vi "SkewedChi2Sampler.vi"(8 "error in":errorcluster caption="entrée d'erreur", 11 "SkewedChi2Sampler":T1={"skewedness"=1.0, "n_components"=100, "random_state"=-1} {"random_state" min=-1}) -> (0 "error out":errorcluster caption="sortie d'erreur", 3 "SkewedChi2Sampler.lvclass":refnum<class "SkewedChi2Sampler.lvclass">)   [LabVIEW 2020]
doc: "Approximates feature map of the “skewed chi-squared” kernel by Monte Carlo approximation of its Fourier transform.\n\nParameters :\n\n- skewedness : float\n“skewedness” parameter of the kernel. Needs to be cross-validated.\n\n- n_components : int\nnumber of Monte Carlo samples per original feature. Equals the dimensionality of the computed feature space.\n\n- random_state : int, RandomState instance or None, optional (default=None=-1)\nPseudo-random number generator to control the generation of the random weights and random offset when fitting the training data. Pass an int for reproducible output across multiple function calls. \n\nMethods : \n\n- Fit : Fit the model with X. Samples random projection according to n_features.\n\nParameters : X : array-like, shape (n_samples, n_features)\n Training data, where n_samples in the number of samples and n_features is the number of features.\n\n- Fit Transform : Fit to data, then transform it. Fits transformer to X and y with optional parameters fit_params and returns a transformed version of X.\n\nParameters : X : {array-like, sparse matrix, dataframe} of shape (n_samples, n_features)\n y : ndarray of shape (n_samples,), default=None\n Target values.\n\nReturns : X_new : ndarray array of shape (n_samples, n_features_new)\nTransformed array.\n\n- Transform : Apply the approximate feature map to X.\n\nParameters : X : array-like, shape (n_samples, n_features)\n New data, where n_samples in the number of samples and n_features is the number of features. All values of X must be strictly greater than “-skewedness”.\n\nReturns : X_new : array-like, shape (n_samples, n_components)"
uses:
  SkewedChi2Sampler.lvclass
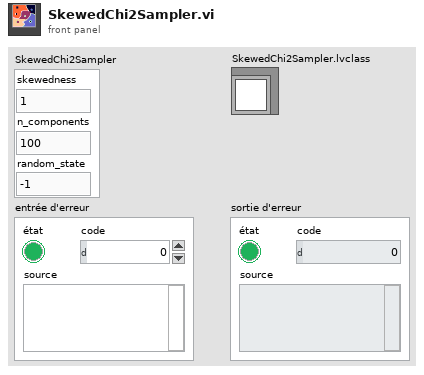
[diagram p1: front panel]
types:
  T1 = cluster{"skewedness":dbl, "n_components":i32, "random_state":i32}
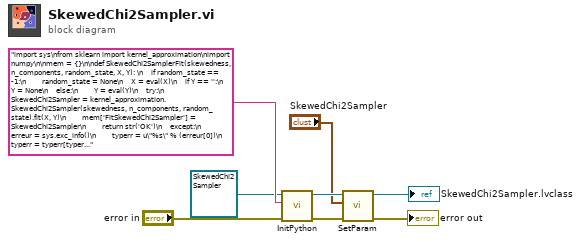
[diagram p0: block diagram]
diagram:
  n1 = call-dynamic "InitPython.vi"("error in (no error)"="error in", "Python Instruction"="import sys\nfrom sklearn import kernel_approximation\nimport numpy\n\nmem = {}\n\ndef SkewedChi2SamplerFit(skewedness, n_components, random_state, X, Y): \n    if random_state == -1:\n        random_state = None\n    X = eval(X)\n    if Y == '':\n        Y = None\n    else:\n        Y = eval(Y)\n    try:\n        SkewedChi2Sampler = kernel_approximation.SkewedChi2Sampler(skewedness, n_components, random_state).fit(X, Y)\n        mem['FitSkewedChi2Sampler'] = SkewedChi2Sampler\n        return str('OK')\n    except:\n        erreur = sys.exc_info()\n        typerr = u\"%s\" % (erreur[0])\n        typerr = typerr[typerr.find(\"'\")+1:typerr.rfind(\"'\")]\n        msgerr = u\"%s\" % (erreur[1])\n        message = str('/!\\\\ {0} : {1}'. format(typerr,msgerr))\n        return message \n\ndef SkewedChi2SamplerFitTransform(skewedness, n_components, random_state, X, Y):\n    if random_state == -1:\n        random_state = None\n    X = eval(X)\n    if Y == '':\n        Y = None\n    else:\n        Y = eval(Y)\n    try:\n        SkewedChi2Sampler = kernel_approximation.SkewedChi2Sampler(skewedness, n_components, random_state).fit_transform(X, Y)\n        SkewedChi2Sampler = SkewedChi2Sampler.tolist()\n        return str(SkewedChi2Sampler)\n    except:\n        erreur = sys.exc_info()\n        typerr = u\"%s\" % (erreur[0])\n        typerr = typerr[typerr.find(\"'\")+1:typerr.rfind(\"'\")]\n        msgerr = u\"%s\" % (erreur[1])\n        message = str('/!\\\\ {0} : {1}'. format(typerr,msgerr))\n        return message \n    \n\ndef SkewedChi2SamplerTransform(skewedness, n_components, random_state, X, Y) :\n    if random_state == -1:\n        random_state = None\n    X = eval(X)\n    if Y == '':\n        Y = None\n    else:\n        Y = eval(Y)\n    try:\n        SkewedChi2Sampler = mem['FitSkewedChi2Sampler'].transform(X, Y)\n        SkewedChi2Sampler = SkewedChi2Sampler.tolist()\n        return str(SkewedChi2Sampler)\n    except:\n        erreur = sys.exc_info()\n        typerr = u\"%s\" % (erreur[0])\n        typerr = typerr[typerr.find(\"'\")+1:typerr.rfind(\"'\")]\n        msgerr = u\"%s\" % (erreur[1])\n        message = str('/!\\\\ {0} : {1}'. format(typerr,msgerr))\n        return message", "Scikit-learn en entrée"=refnum<class "SkewedChi2Sampler.lvclass"> refnum ("SkewedChi2Sampler.lvclass")) -> ("error out"=w6:errorcluster, "Scikit-learn en sortie"=w5:refnum<class "SkewedChi2Sampler.lvclass">)  [unwired: 7 in]
  n2 = call-dynamic "SetParam.vi"("error in (no error)"=w6, "SkewedChi2Sampler"="SkewedChi2Sampler", "SkewedChi2Sampler.lvclass"=w5) -> ("error out"=→"error out":errorcluster, "SkewedChi2Sampler.lvclass"=→"SkewedChi2Sampler.lvclass":refnum<class "SkewedChi2Sampler.lvclass">)  [unwired: 7 in]
